vi "Configure Surge-Drop Start Time.vi"(0 "VISA resource name":refnum<visa-resource-name>, 5 "Surge Drop Start Time (0 ms)":dbl min=0.0 max=99.0, 11 "error in (no error)":errorcluster) -> (4 "VISA resource name out":refnum<visa-resource-name>, 15 "error out":errorcluster)   [LabVIEW 2020, in "eec 6700.lvlib"]
doc: "Sets <B>Surge drop start time</B> of the power source instrument.\n\n<B>Range</B> : \nIf Surge Drop Continuous = ON : 0 ~ 20ms\nIf Surge Drop Continuous = OFF : 0 ~ 99ms\n\nSD-Site setting gives user the flexibility to program the specific point of the sine wave to initialize the surge or the drop voltage. \n\nFor example:\n\nConsider a sine wave with a time period of 1 second (Freq = 1 Hz). \nIf SD-Site is configured @ 500 milliseconds the surge or the drop voltage will occur at the halfway point (500 millisecond) of the sine wave or at the 180º point."
uses:
  <instrlib>/EEC6700LV-driver/eec 6700.lvlib
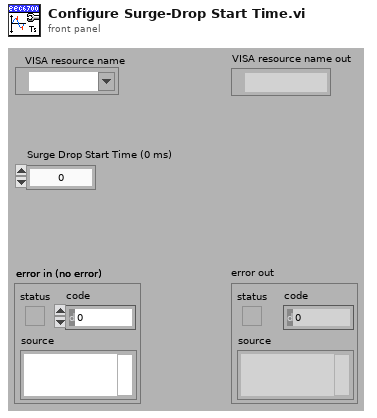
[diagram p1: front panel]
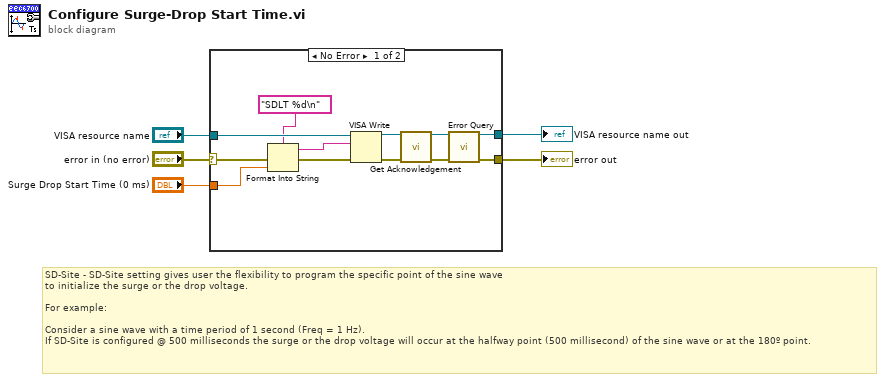
[diagram p0: block diagram]
diagram:
  # "SD-Site - SD-Site setting gives user the flexibility to program the specific point of the sine wave \nto initialize the surge or the drop voltage. \n\nFor example:\n\nConsider a sine wave with a time period of 1 second (Freq = 1 Hz). \nIf SD-Site is configured @ 500 milliseconds the surge or the drop voltage will occur at the halfway point (500 millisecond) of the sine wave or at the 180º point."
  n1 = case shown="No Error" "error in (no error)" {
    selector: "error in (no error)" -> [w11 w19]
    tunnel: [w12 w19] -> w5
    tunnel: [w13 w18] -> w4
    tunnel: "VISA resource name" -> [w17 w18]
    tunnel: "Surge Drop Start Time (0 ms)" -> [w16 _]
    frame No Error {
      n2 = Format Into String(format string="SDLT %d\n" ("Command"), error in=w11, w16) -> (resulting string=w15:string, error out=w10:errorcluster)  [unwired: 1 in]
      n3 = VISA Write(VISA resource name=w17, write buffer=w15, error in (no error)=w10) -> (VISA resource name out=w6:refnum<visa-resource-name>, error out=w9:errorcluster)  [unwired: 1 out]
      n4 = call <instrlib>:"Get Acknowledgement.vi"("VISA resource name"=w6, "error in (no error)"=w9) -> ("VISA resource name out"=w7:refnum<visa-resource-name>, "error out"=w8:errorcluster)  [unwired: 12 in]
      n5 = call <instrlib>:"Error Query.vi"("VISA resource name"=w7, "error in (no error)"=w8) -> ("VISA resource name out"=w13:refnum<visa-resource-name>, "error out"=w12:errorcluster)  [unwired: 10 in, 2 out]
    }
    frame Error {
    }
  }
  "error out" <- w5
  "VISA resource name out" <- w4
